vi "CountsTillNextCommonTrigger.vi"(8 "error in (no error)":errorcluster, 10 "MasterTriggerCounter":i64=2147483647, 11 "BME_DG_System in":refnum<class "BME_DG_System.lvclass">) -> (0 "error out":errorcluster, 1 "LeastCommonMult":i64, 2 "CountsRemains":i64, 3 "BME_DG_System out":refnum<class "BME_DG_System.lvclass">)   [LabVIEW 2009, in "POLARIS BME DG.lvlib" / "BME_DG_System.lvclass"]
doc: "Calculates trigger counts till next common shot at all channels.\n\n\n\n---------------\n\nauthor: Alexander Kessler, Helmholtz-Institut-Jena \nmaintainer: Alexander Kessler: alexander.kessler@uni-jena.de\n\n\nLicense Agreement for this software:\n\nCopyright (C)\nHelmholtz-Institut-Jena\nFröbelsteg 3\n07743 Jena\nGermany\n\nContact: alexander.kessler@uni-jena.de\n\nThis program is free software; you can redistribute it and/or modify it under the terms of the GNU General Public License as published by the Free Software Foundation; either version 2 of the license, or (at your option) any later version.\n\nThis program is distributed in the hope that it will be useful, but WITHOUT ANY WARRANTY; without even the implied warranty of MERCHANTABILITY or FITNESS FOR A PARTICULAR PURPOSE. See the GNU General License for more details (http://www.gnu.org)."
uses:
  BME_DG_System.lvclass
  BME_DG_System.lvclass/BME_DG_System.ctl
  POLARIS BME DG.lvlib
  BME_DG_Base/BME_DG_Base.lvclass
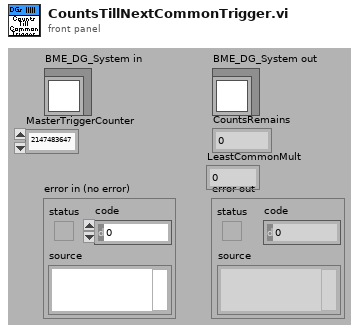
[diagram p1: front panel]
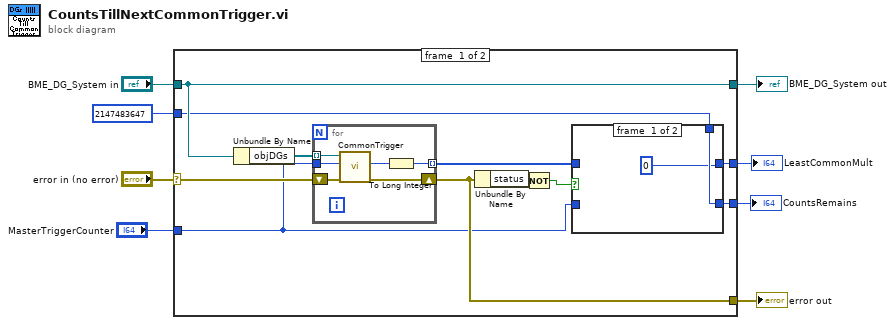
[diagram p0: block diagram]
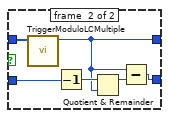
[diagram p2: hidden frame]
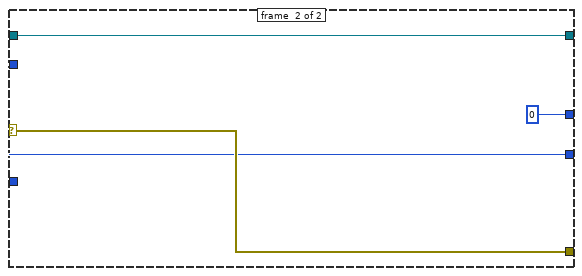
[diagram p3: hidden frame]
diagram:
  n1 = case shown="No Error" "error in (no error)" {
    selector: "error in (no error)" -> [w16 w37]
    tunnel: [w13 w37] -> w7
    tunnel: [w19 w36] -> w5
    tunnel: "BME_DG_System in" -> [w19 w36]
    tunnel: [w14 w35] -> w3
    tunnel: i64 2147483647 -> [w12 w35]
    tunnel: [w11 0] -> w2
    tunnel: "MasterTriggerCounter" -> [w9 _]
    frame #0 {
      n2 = Unbundle By Name(w19) -> ("objDGs"=w18:refnum<class "BME_DG_Base.lvclass">[])
      n3 = for {
        tunnel: w18 -> [w33] mode=indexing
        tunnel: [w28] -> w17 mode=indexing
        shift-right: [w30] -> w13
        shift-left: w16 -> [w31]
        tunnel: w9 -> [w29]
        n4 = call "CommonTrigger.vi"("error in (no error)"=w31, "MasterTriggerCounter"=w29, "BME_DG_Base in"=w33) -> ("error out"=w30:errorcluster, "TriggerModuloLCMult"=w32:i64)  [unwired: 5 in, 2 out]
        n5 = To Long Integer(number=w32) -> (32bit integer=w28:i32)
      }
      n6 = Unbundle By Name(w13) -> ("status"=w15:bool)
      n7 = Not(x=w15) -> (.not. x?=w10:bool)
      n8 = case shown="True" w10 {
        tunnel: w17 -> [_ w27]
        tunnel: w9 -> [_ w26]
        tunnel: [w21 w23] -> w14
        tunnel: w12 -> [w21 _]
        tunnel: [0 w22] -> w11
        frame #0 {
        }
        frame #1 {
          n9 = call "TriggerModuloLCMultiple.vi"("TriggerModulos"=w27) -> ("LeastCommonMult"=w22:i64)  [unwired: 10 in]
          n10 = Decrement(x=w26) -> (x-1=w25:i64)
          n11 = Quotient & Remainder(x=w25, y=w22) -> (x-y*floor(x/y)=w24:i64)  [unwired: 1 out]
          n12 = Subtract(x=w22, y=w24) -> (x-y=w23:i64)
        }
      }
    }
    frame #1 {
    }
  }
  "error out" <- w7
  "BME_DG_System out" <- w5
  "CountsRemains" <- w3
  "LeastCommonMult" <- w2
